vi "ExecPratAulaWhileCase.vi"() -> ()   [LabVIEW 2020]
panel:
  in  "Numeric":fxp<+/-,64,32>
  in  "stop 2":bool
  out "(i) 2":i32
  in  "milliseconds to wait 2":u32
  in  "Farhenreit 2":dbl(slide) scale=0.0..300.0
  out "Celsius 2":dbl(slide) scale=-200.0..100.0
  in  "Boolean":bool
  out "Celsius":dbl(slide) scale=-200.0..100.0
  in  "Farhenreit":dbl(slide) scale=0.0..300.0
  in  "milliseconds to wait":u32
  out "(i)":i32
  in  "stop":bool
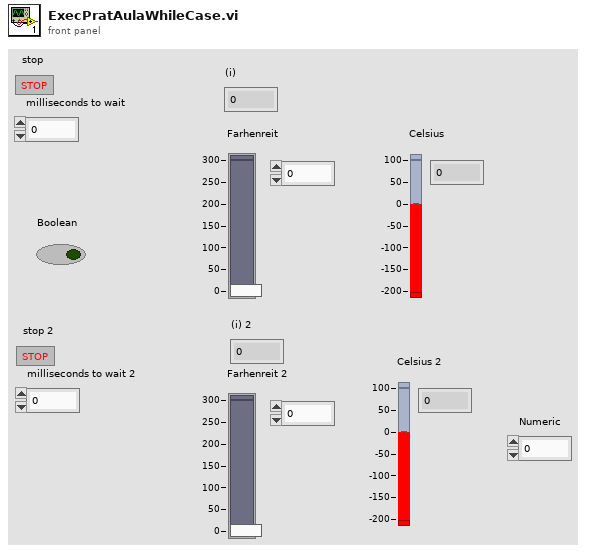
[diagram p1: front panel]
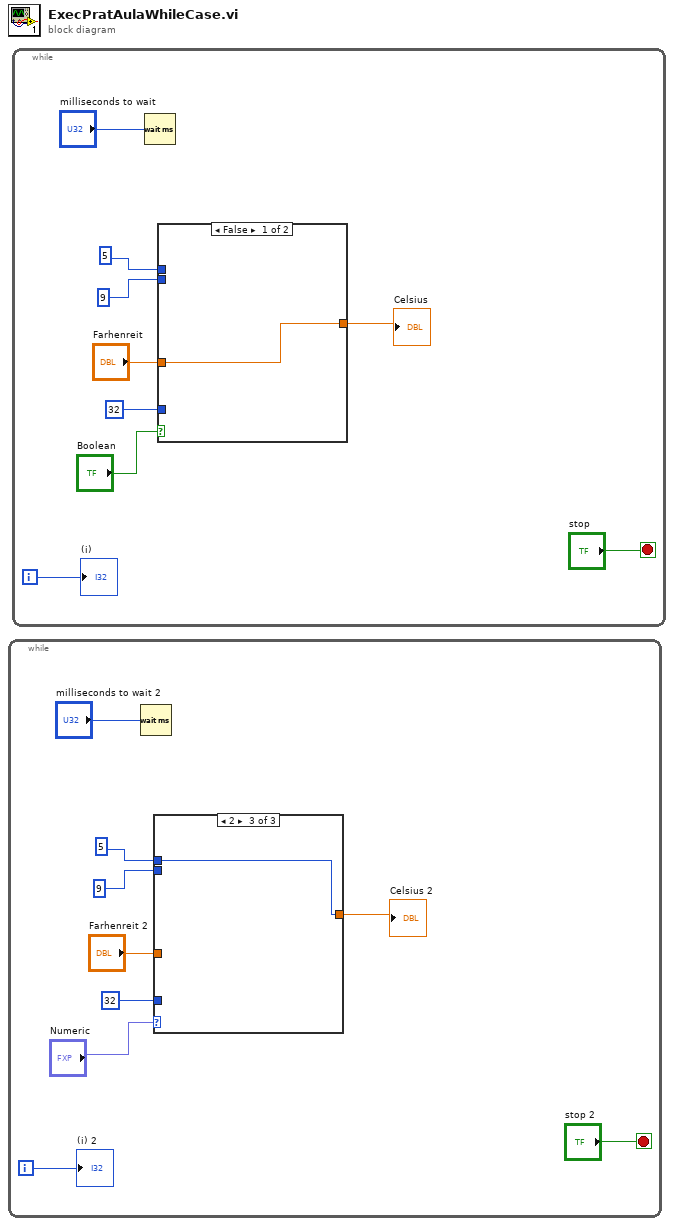
[diagram p0: block diagram]
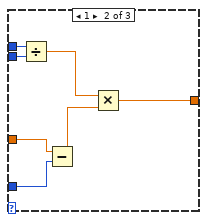
[diagram p3: hidden frame]
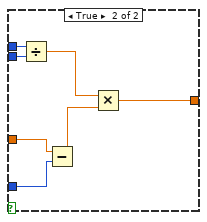
[diagram p4: hidden frame]
diagram:
  n1 = while {
    i -> [w8]
    stop <- "stop 2" stop-if-true
    n2 = Wait (ms)(milliseconds to wait="milliseconds to wait 2") -> ()  [unwired: 1 out]
    n3 = case shown="2" "Numeric" {
      tunnel: 5 -> [_ w17 w18]
      tunnel: 9 -> [_ w16 _]
      tunnel: "Farhenreit 2" -> [w10 w15 _]
      tunnel: 32 -> [_ w14 _]
      tunnel: [w10 w11 w18] -> w2
      frame 0, Default {
      }
      frame 1 {
        n4 = Divide(x=w17, y=w16) -> (x/y=w13:dbl)
        n5 = Subtract(x=w15, y=w14) -> (x-y=w12:dbl)
        n6 = Multiply(x=w13, y=w12) -> (x*y=w11:dbl)
      }
      frame 2 {
      }
    }
    "Celsius 2" <- w2
    "(i) 2" <- w8
  }
  n7 = while {
    i -> [w26]
    stop <- "stop" stop-if-true
    n8 = Wait (ms)(milliseconds to wait="milliseconds to wait") -> ()  [unwired: 1 out]
    n9 = case shown="False" "Boolean" {
      tunnel: 5 -> [_ w35]
      tunnel: 9 -> [_ w34]
      tunnel: "Farhenreit" -> [w28 w33]
      tunnel: 32 -> [_ w32]
      tunnel: [w28 w29] -> w20
      frame False {
      }
      frame True {
        n10 = Divide(x=w35, y=w34) -> (x/y=w31:dbl)
        n11 = Subtract(x=w33, y=w32) -> (x-y=w30:dbl)
        n12 = Multiply(x=w31, y=w30) -> (x*y=w29:dbl)
      }
    }
    "Celsius" <- w20
    "(i)" <- w26
  }
